vi "MAIN LIST Layouts.vi"(8 "error in (no error)":errorcluster, 11 "Domino Laser module Class in":refnum<class "Domino Laser module Class.lvclass">) -> (0 "error out":errorcluster, 3 "Domino Laser module Class out":refnum<class "Domino Laser module Class.lvclass">)   [LabVIEW 2024, in "Domino LM.lvlib" / "Domino Laser module Class.lvclass"]
uses:
  CTRLS/Domino Laser module Class.lvclass
  CTRLS/Domino Laser module Class.lvclass/Domino Laser module Class.ctl
  <userlib>/_OpenG.lib/string/string.llb/openg_string.lvlib
panel:
  out "Array":string[](array[string])
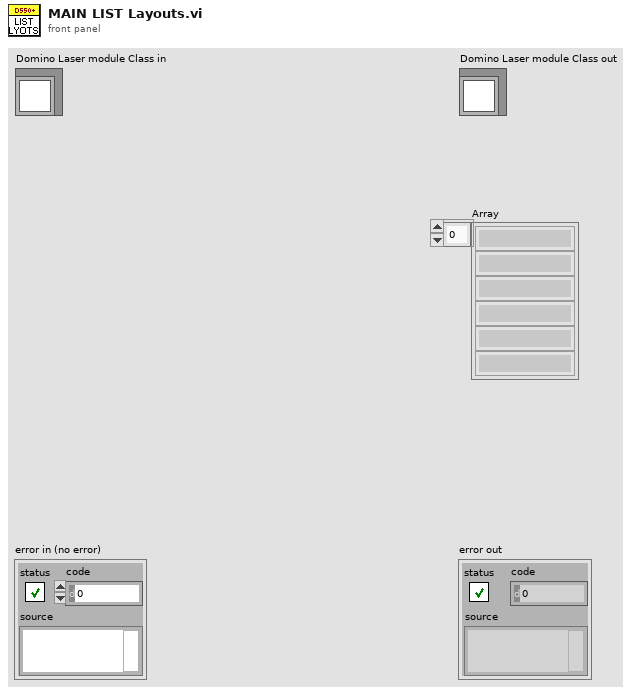
[diagram p1: front panel]
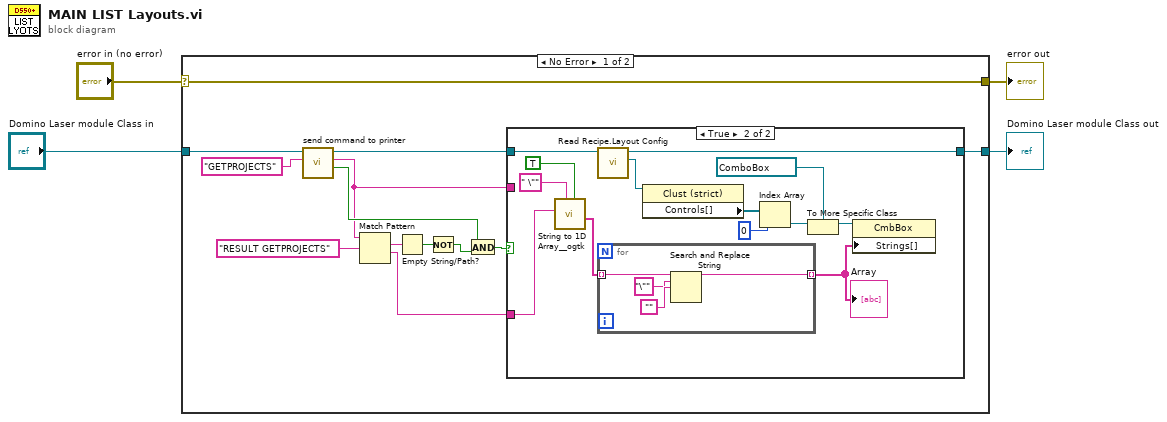
[diagram p0: block diagram]
diagram:
  n1 = case shown="No Error" "error in (no error)" {
    selector: "error in (no error)" -> [w17 w37]
    tunnel: [w17 w37] -> w3
    tunnel: [w10 w36] -> w1
    tunnel: "Domino Laser module Class in" -> [w16 w36]
    frame No Error {
      n2 = call "send command to printer.vi"("command to be sent"="GETPROJECTS", "Domino Laser module Class in"=w16) -> ("Command Excuted succeddfully?"=w9:bool, "Recived message"=w5:string, "Domino Laser module Class out"=w11:refnum<class "Domino Laser module Class.lvclass">)  [unwired: 6 in, 1 out]
      n3 = Match Pattern(string=w5, regular expression="RESULT GETPROJECTS") -> (match substring=w13:string, after substring=w12:string)  [unwired: 1 in, 2 out]
      n4 = Empty String/Path?(string/path=w13) -> (empty?=w7:bool)
      n5 = Not(x=w7) -> (.not. x?=w6:bool)
      n6 = And(x=w9, y=w6) -> (x .and. y?=w8:bool)
      n7 = case shown="True" w8 {
        tunnel: w12 -> [_ w30]
        tunnel: w11 -> [w18 w23]
        tunnel: [w18 w22] -> w10
        tunnel: w5 -> [_ _]
        frame False {
        }
        frame True {
          n8 = call <userlib>:"String to 1D Array__ogtk.vi"("ignore duplicate delimiters? (F=No)"=TRUE, "delimiter (Tab)"=" \"", "string"=w30) -> ("Array of Strings"=w28:string[])  [unwired: 8 in]
          n9 = call "Read Recipe.Layout Config.vi"("Domino Laser module Class in"=w23) -> ("Recipe.Layout Config"=w21:refnum<vi>, "Domino Laser module Class out"=w22:refnum<class "Domino Laser module Class.lvclass">)  [unwired: 8 in, 1 out]
          n10 = for {
            tunnel: w28 -> [w33] mode=indexing
            tunnel: [w32] -> w20 mode=indexing
            n11 = Search and Replace String(input string=w33, search string="\"", replace string="") -> (result string=w32:string)  [unwired: 5 in, 3 out]
          }
          "Array" <- w20
          n12 = property class="Clust (strict)"(reference=w21) -> ("Controls[]"=w24:refnum<vi>[])  [unwired: 1 in, 2 out]
          n13 = Index Array(array=w24, index=0) -> (element=w25:refnum<vi>)
          n14 = To More Specific Class(target class=refnum<vi> refnum ("Layout File"), reference=w25) -> (specific class reference=w26:refnum<vi>)  [unwired: 1 in, 1 out]
          n15 = property class="CmbBox"(reference=w26, "Strings[]"=w20) -> ()  [unwired: 1 in, 2 out]
        }
      }
    }
    frame Error {
    }
  }
  "error out" <- w3
  "Domino Laser module Class out" <- w1
